vi "PathPlanner_FieldUtil_SymmetryType.vi"() -> (3 "PathPlanner_FieldSymmetry":T1)   [LabVIEW 2019, in "PathPlanner24.lvlib"]
doc: "The type of symmetry for the current field\n\nInputs:\n -- <none>\n\nOutputs:\n -- FieldSymmetryType - The type of symmetry for the current field"
uses:
  PathPlanner24.lvlib
  ENum/PathPlanner_FieldSymmetry_ENUM.ctl
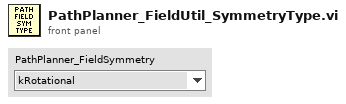
[diagram p1: front panel]
types:
  T1 = typedef "PathPlanner24.lvlib/PathPlanner_FieldSymmetry_ENUM.ctl" = enum16{"kRotational", "kMirrored"}
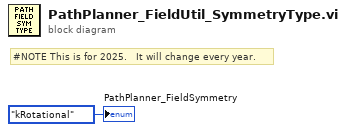
[diagram p0: block diagram]
diagram:
  # "#NOTE This is for 2025.   It will change every year."
  "PathPlanner_FieldSymmetry" <- PathPlanner_FieldSymmetry_ENUM."kRotational" ("PathPlanner_FieldSymmetry")
